vi "Variant.vi"() -> (0 "error out":errorcluster)   [LabVIEW 2020, in "Memory Manager Tests.lvlib" / "Malleable Type Tests.lvclass"]
uses:
  Malleable Type Tests.lvclass
  Source/Classes/Pointer/Pointer.lvclass
  f519fe4c-294f-4b55-907f-fdec5b18c042.vi
  Source/Classes/Pointer/Check Null Pointer.vi
  Source/Classes/Pointer/Get Size.vi
  Source/Classes/Pointer/Get Address.vi
  <vilib>/Utility/error.llb/Error Cluster From Error Code.vi
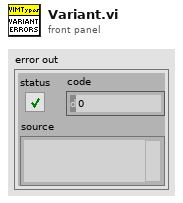
[diagram p1: front panel]
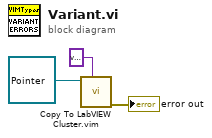
[diagram p0: block diagram]
diagram:
  n1 = call "Copy To LabVIEW Cluster.vim"("Type"=variant, "Pointer in"=refnum<class "Pointer.lvclass"> refnum) -> ("error out"=→"error out":errorcluster)  [unwired: 7 in, 2 out]
